vi "Remove Duplicates from 1D String Array.vi"(1 "String Array In":string[](array[string])) -> (0 "String Array Out":string[](array[string]))   [LabVIEW 2016, in "SLL Table.lvclass"]
uses:
  SLL Table.lvclass
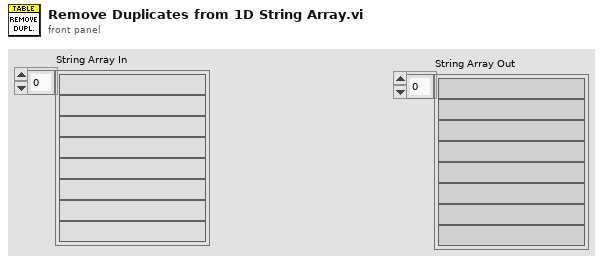
[diagram p1: front panel]
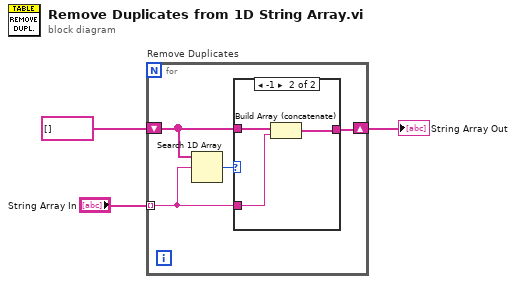
[diagram p0: block diagram]
diagram:
  n1 = for "Remove Duplicates" {
    tunnel: "String Array In" -> [w5] mode=indexing
    shift-right: [w4] -> w1
    shift-left: string[] [] -> [w6]
    n2 = Search 1D Array(1D array=w6, element=w5) -> (index of element=w7:i32)  [unwired: 1 in]
    n3 = case shown="-1" w7 {
      tunnel: w6 -> [w8 w11]
      tunnel: w5 -> [_ w10]
      tunnel: [w8 w9] -> w4
      frame 0, Default {
      }
      frame -1 {
        n4 = Build Array (concatenate)(w11, w10) -> (w9:string[])
      }
    }
  }
  "String Array Out" <- w1
